vi "SwissSPAD Live_Update Settings & Control.vi"(8 "Error In":errorcluster, 9 "Value":variant, 10 "Sender":string="SS2 DAQ", 11 "CtlRef":refnum<vi>) -> (0 "Error Out":errorcluster, 2 "Control Label":string)   [LabVIEW 2021]
uses:
  SwissSPAD Live_Settings Event.ctl
  SwissSPAD Live_Settings Window Messages.ctl
  SwissSPAD Live_Settings List.ctl
  Notebook/Notebook.lvlib
  Rich Text Box/Rich Text Box.lvlib
  Variant/Variant to Data/Variant to Data.lvlib
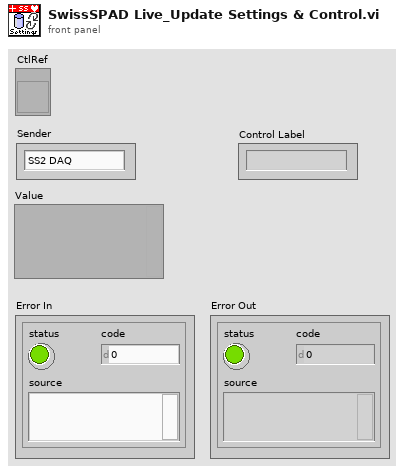
[diagram p1: front panel]
types:
  T1 = typedef "SwissSPAD Live_Settings List.ctl" = enum16{"FPGA:Bottom Half", "FPGA:Top Half", "FPGA:Bottom Bitfile Path", "FPGA:Top Bitfile Path", "FPGA:Bottom Bitstream Version", "FPGA:Top Bitstream Version", "FPGA:Auto Reset FPGA", "FPGA:Bottom FPGA Serial Number", "FPGA:Top FPGA Serial Number", "FPGA:Detector PCB Version", "Acquisition Parameters:Microlens", "Acquisition Parameters:SS2 DAQ Parameters", "Acquisition Parameters:Gate Configuration Array", "Acquisition Parameters:SS3 DAQ Parameters", "Acquisition Parameters:Buffer Size (# 8-bit Gates)", "File Information:File Information", "File Information:# Datasets in Series", "File Information:Scrambled File Flag", "File Information:SS3 Gate Slip Correction", "File Information:SS3 Hot Pixel Mismatch Detection", "File Information:Delay between Datasets", "File Information:Save Sum of All Gates Preview", "Image Parameters:Image ROI Information", "Image Parameters:Image Binning Options", "Image Parameters:SS3 Displayed Image", "Image Parameters:Image Display Options", "Image Parameters:Use Histogram Cursors", "Image Parameter:FPGA Data to Display", "UI Settings:Histogram Bins Number", "UI Settings:Histogram Bin Size", "UI Settings:Use Image Display Options", "UI Settings:Verbose Settings", "UI Settings:Verbose Saving"}
  T2 = typedef "SwissSPAD Live_Settings Event.ctl" = cluster{"Settings Message":T3, "Sender":string, "Control Label":string, "Data":variant}
  T3 = typedef "SwissSPAD Live_Settings Window Messages.ctl" = enum16{"Idle", "Subscribe", "Unsubscribe", "Refresh Parameter", "Refresh All Parameters", "Quit"}
  T4 = typedef "Rich Text Box.lvlib/Text Formatting.ctl" = cluster{"Font":string, "Text Color":T5, "Text Background Color":T5, "Text Style":enum16{"Regular", "Bold", "Italic", "Underline", "Strikeout"}, "Font Size (Points)":dbl, "Text Alignment":i32}
  T5 = typedef "Rich Text Box.lvlib/Text Colors.ctl" = enum16{"Unchanged", "Black", "Blue", "Brown", "Gray", "Green", "Orange", "Pink", "Red", "White"}
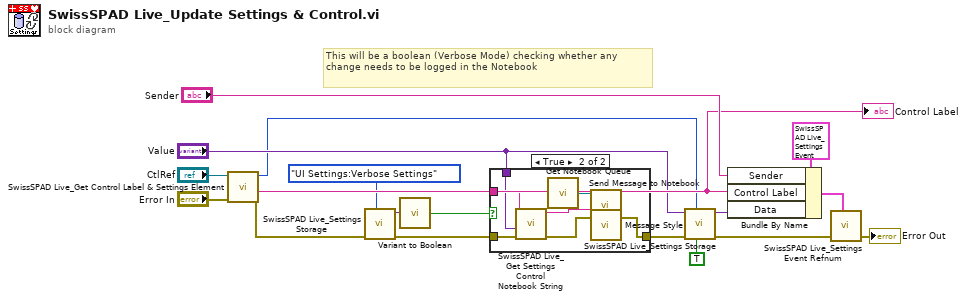
[diagram p0: block diagram]
diagram:
  # "This will be a boolean (Verbose Mode) checking whether any change needs to be logged in the Notebook"
  n1 = call "SwissSPAD Live_Get Control Label & Settings Element.vi"("Error In"="Error In", "CtlRef"="CtlRef") -> ("Error Out"=w10:errorcluster, "Control Label"=w8:string, "Settings Element"=w5:T1)  [unwired: 7 in]
  "Control Label" <- w8
  n2 = call "SwissSPAD Live_Settings Storage.vi"("Settings List"=SwissSPAD_Live_Settings_List."UI Settings:Verbose Settings", "Error In"=w10) -> ("Error Out"=w3:errorcluster, "Variant Data out"=w2:variant)  [unwired: 8 in]
  n3 = call "Variant to Boolean.vi"("Variant"=w2) -> ("Value"=w4:bool)  [unwired: 8 in]
  n4 = case shown="True" w4 {
    tunnel: w8 -> [_ w27]
    tunnel: "Value" -> [_ w26]
    tunnel: w3 -> [w19 w25]
    tunnel: [w19 w21] -> w9
    frame False {
    }
    frame True {
      n5 = call "SwissSPAD Live_Get Settings Control Notebook String.vi"("error in (no error)"=w25, "Value"=w26, "Control Label"=w27) -> ("error out"=w22:errorcluster, "Notebook String"=w23:string)  [unwired: 7 in]
      n6 = call "Get Notebook Queue.vi"() -> ("Notebook Queue"=w24:refnum<queue>)  [unwired: 9 in]
      n7 = call "Message Style.vi"() -> ("Message Formatting"=w20:T4)
      n8 = call "Send Message to Notebook.vi"("Text Formatting"=w20, "Error In"=w22, "Message"=w23, "Notebook Queue"=w24) -> ("Error Out"=w21:errorcluster)  [unwired: 4 in, 1 out]
    }
  }
  n9 = call "SwissSPAD Live_Settings Storage.vi"("Set/Get(F)"=TRUE ("Get(F)/Set"), "Settings List"=w5, "Error In"=w9, "Variant Data in"="Value") -> ("Error Out"=w14:errorcluster, "Variant Data out"=w6:variant)  [unwired: 6 in]
  n10 = Bundle By Name(cluster=T2 {"Settings Message"=enum."Refresh Parameter", "Sender"="", "Control Label"="", "Data"=variant}, "Sender"="Sender", "Control Label"=w8, "Data"=w6) -> (w12:T2)
  n11 = call "SwissSPAD Live_Settings Event Refnum.vi"("Settings Event"=w12, "Error In"=w14) -> ("Error Out"=→"Error Out":errorcluster)  [unwired: 6 in, 1 out]
